vi "WriteTestingDB.vi"(6 "AuthCode":string, 7 "PartN":string="1805", 8 "error in":errorcluster caption="错误输入", 9 "Imei":string, 10 "ICCID":string, 11 "SN":string) -> (0 "error out":errorcluster caption="错误输出", 3 "ReportStrA":string)   [LabVIEW 2013]
panel:
  out "连接的字符串":string
  out "Certid":string
  out "TUID":string
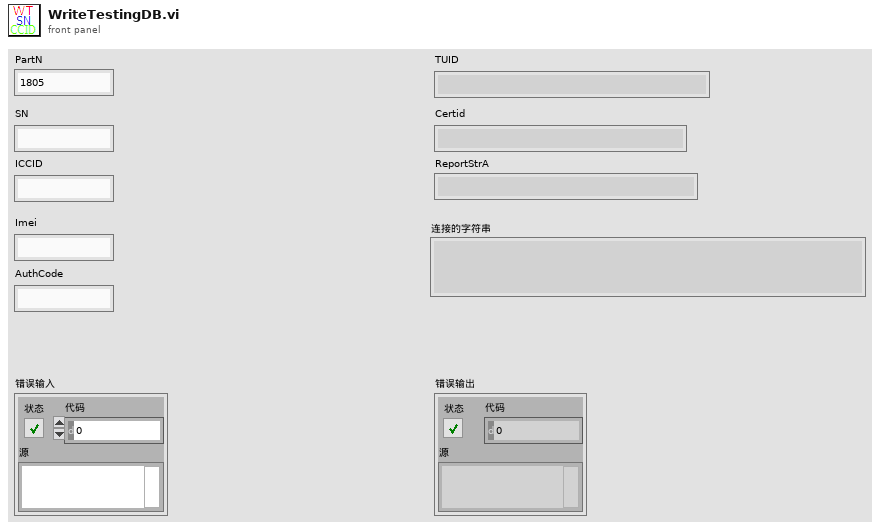
[diagram p1: front panel]
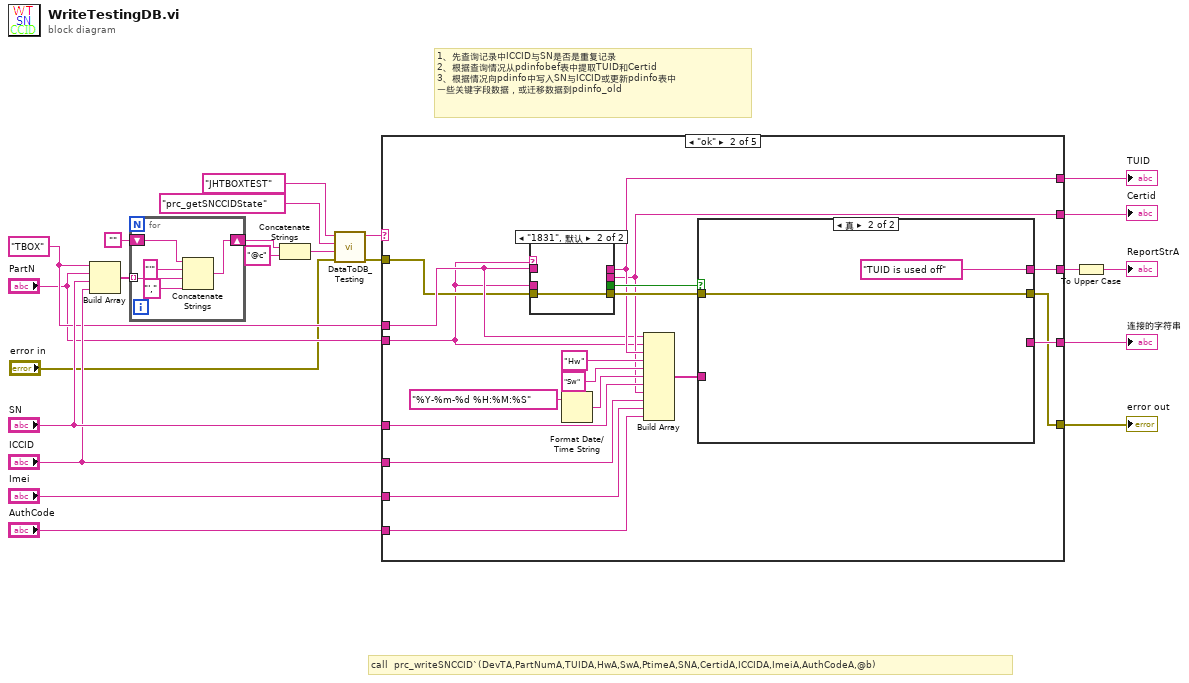
[diagram p0: block diagram]
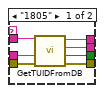
[diagram p3: hidden frame]
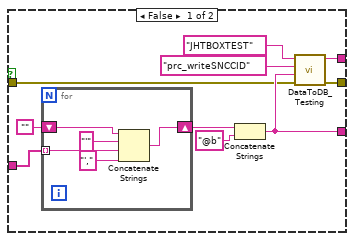
[diagram p4: hidden frame]
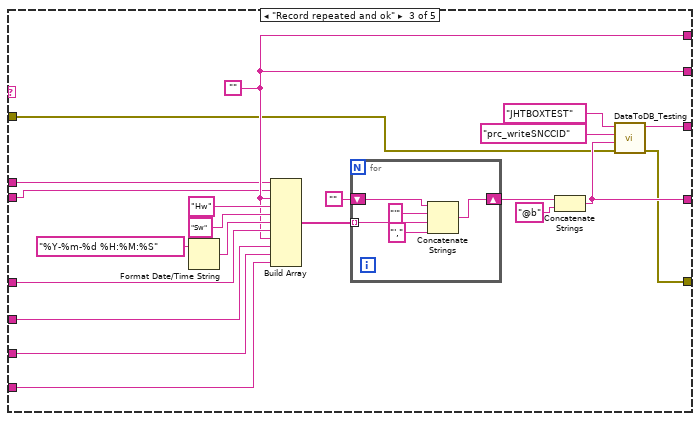
[diagram p5: hidden frame]
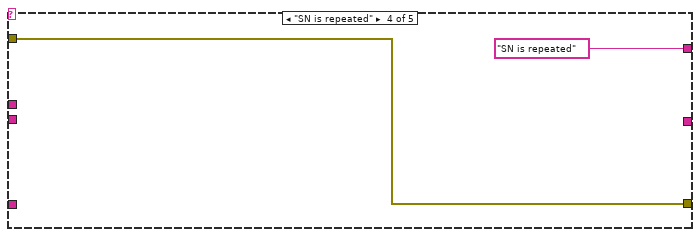
[diagram p6: hidden frame]
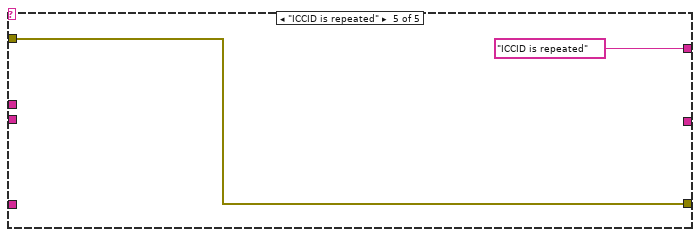
[diagram p7: hidden frame]
diagram:
  w6 = "TBOX" ("DeviceType")
  # "1、先查询记录中ICCID与SN是否是重复记录\n2、根据查询情况从pdinfobef表中提取TUID和Certid\n3、根据情况向pdinfo中写入SN与ICCID或更新pdinfo表中\n一些关键字段数据，或迁移数据到pdinfo_old"
  # "call  prc_writeSNCCID`(DevTA,PartNumA,TUIDA,HwA,SwA,PtimeA,SNA,CertidA,ICCIDA,ImeiA,AuthCodeA,@b)"
  n1 = Build Array(w6, "PartN", "SN", "ICCID") -> (w15:string[])
  n2 = for {
    shift-right: [w26] -> w14
    shift-left: "" -> [w27]
    tunnel: w15 -> [w23] mode=indexing
    n3 = Concatenate Strings(w27, "'", w23, "',") -> (w26:string)
  }
  n4 = Concatenate Strings(w14, "@c" ("字符串")) -> (w12:string)
  n5 = call "DataToDB_Testing.vi"("error in (no error)"="error in", "all string"=w12, "Procedure name"="prc_getSNCCIDState" ("DSN name"), "DSN name"="JHTBOXTEST") -> ("error out"=w3:errorcluster, "ReportStrA"=w9:string)  [unwired: 6 in]
  n6 = case shown="\"ok\"" w9 {
    tunnel: [_ w47 w93 _ _] -> w22
    tunnel: [_ w46 w92 "SN is repeated" "ICCID is repeated"] -> w21
    tunnel: "Imei" -> [_ w40 w86 _ _]
    tunnel: "AuthCode" -> [_ w39 w85 _ _]
    tunnel: "SN" -> [_ w37 w84 _ _]
    tunnel: "ICCID" -> [_ w36 w83 _ _]
    tunnel: [_ w34 w82 _ _] -> w8
    tunnel: [_ w33 w82 _ _] -> w7
    tunnel: w6 -> [_ w32 w76 _ _]
    tunnel: "PartN" -> [_ w29 w75 _ _]
    tunnel: w3 -> [w28 w31 w74 w99 w101]
    tunnel: [w28 w30 w73 w99 w101] -> w2
    frame "假", Default {
    }
    frame "ok" {
      n7 = case shown="\"1831\", 默认" w29 {
        tunnel: [w54 w55] -> w38
        tunnel: [w53 _] -> w35
        tunnel: [w52 _] -> w34
        tunnel: [w51 _] -> w33
        tunnel: w32 -> [w50 _]
        tunnel: w29 -> [w49 _]
        tunnel: w31 -> [w48 w55]
        frame "1805" {
          n8 = call "GetTUIDFromDB.vi"("error in"=w48, "PartNumber"=w49, "DeviceType"=w50) -> ("error out"=w54:errorcluster, "Empty？"=w53:bool, "Certid"=w51:string, "TUID"=w52:string)  [unwired: 5 in]
        }
        frame "1831", Default {
        }
      }
      n9 = Format Date/Time String(time format string (%c)="%Y-%m-%d %H:%M:%S" ("Procedure name")) -> (date/time string=w42:string)  [unwired: 2 in]
      n10 = Build Array(w32, w29, w34, "Hw" ("DeviceType"), "Sw" ("DeviceType"), w42, w37, w33, w36, w40, w39) -> (w41:string[])
      n11 = case shown="真" w35 {
        tunnel: [w60 _] -> w47
        tunnel: [w59 "TUID is used off"] -> w46
        tunnel: w41 -> [w58 _]
        tunnel: w38 -> [w57 w71]
        tunnel: [w56 w71] -> w30
        frame False {
          n12 = for {
            shift-right: [w69] -> w64
            shift-left: "" -> [w70]
            tunnel: w58 -> [w66] mode=indexing
            n13 = Concatenate Strings(w70, "'", w66, "',") -> (w69:string)
          }
          n14 = Concatenate Strings(w64, "@b") -> (w60:string)
          n15 = call "DataToDB_Testing.vi"("error in (no error)"=w57, "all string"=w60, "Procedure name"="prc_writeSNCCID", "DSN name"="JHTBOXTEST") -> ("error out"=w56:errorcluster, "ReportStrA"=w59:string)  [unwired: 6 in]
        }
        frame True {
        }
      }
    }
    frame "Record repeated and ok" {
      w82 = ""
      n16 = Format Date/Time String(time format string (%c)="%Y-%m-%d %H:%M:%S" ("Procedure name")) -> (date/time string=w88:string)  [unwired: 2 in]
      n17 = Build Array(w76, w75, w82, "Hw" ("DeviceType"), "Sw" ("DeviceType"), w88, w84, w82, w83, w86, w85) -> (w87:string[])
      n18 = for {
        shift-right: [w97] -> w80
        shift-left: "" -> [w98]
        tunnel: w87 -> [w94] mode=indexing
        n19 = Concatenate Strings(w98, "'", w94, "',") -> (w97:string)
      }
      n20 = Concatenate Strings(w80, "@b") -> (w93:string)
      n21 = call "DataToDB_Testing.vi"("error in (no error)"=w74, "all string"=w93, "Procedure name"="prc_writeSNCCID", "DSN name"="JHTBOXTEST") -> ("error out"=w73:errorcluster, "ReportStrA"=w92:string)  [unwired: 6 in]
    }
    frame "SN is repeated" {
    }
    frame "ICCID is repeated" {
    }
  }
  "连接的字符串" <- w22
  "TUID" <- w8
  "Certid" <- w7
  "error out" <- w2
  n22 = To Upper Case(1:w21) -> (0:→"ReportStrA":string)
